vi "process vision.vi"(8 "?":errorcluster, 11 "Processed Image":T1(plugin-control)) -> (2 "Annotated Image Out":T1(plugin-control), 3 "Processed Image Out":T1(plugin-control))   [LabVIEW 2015]
uses:
  <vilib>/vision/NI_Vision_Development_Module.lvlib
panel:
  out "output cluster":cluster{dbl[], dbl[], dbl[]}
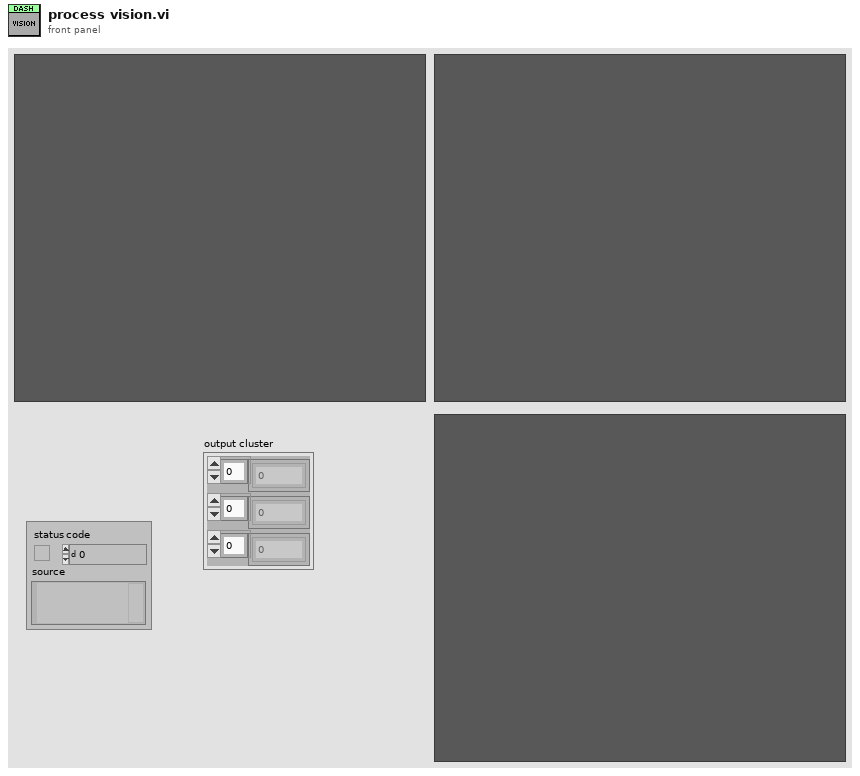
[diagram p1: front panel]
types:
  T1 = typedef "IMAQ Image.ctl" = refnum<image>
  T2 = typedef "Image Type" = u32
  T3 = cluster{"Desired Font (Application)":enum16{"User-specified Font", "Application Font", "System Font", "Dialog Font"}, "[User-specified Font]":cluster{"Font Name":string, "Size":i16, "Strikeout?":bool, "Italic?":bool, "Underline?":bool, "Outline?":bool, "Shadow?":bool, "Bold?":bool, "Rotation Angle":dbl}, "Horizontal Alignment":i16, "Vertical Alignment":i16}
  T4 = cluster{"Left":i32, "Top":i32, "Right":i32, "Bottom":i32}
  T5 = cluster{"Area":dbl, "Number of Holes":dbl, "Bounding Rect":cluster{"Left":dbl, "Top":dbl, "Right":dbl, "Bottom":dbl}, "Center of Mass":cluster{"X":dbl, "Y":dbl}, "Orientation":dbl, "Dimensions":cluster{"Width":dbl, "Height":dbl}}[]
  T6 = cluster{"Left":dbl, "Top":dbl, "Right":dbl, "Bottom":dbl}
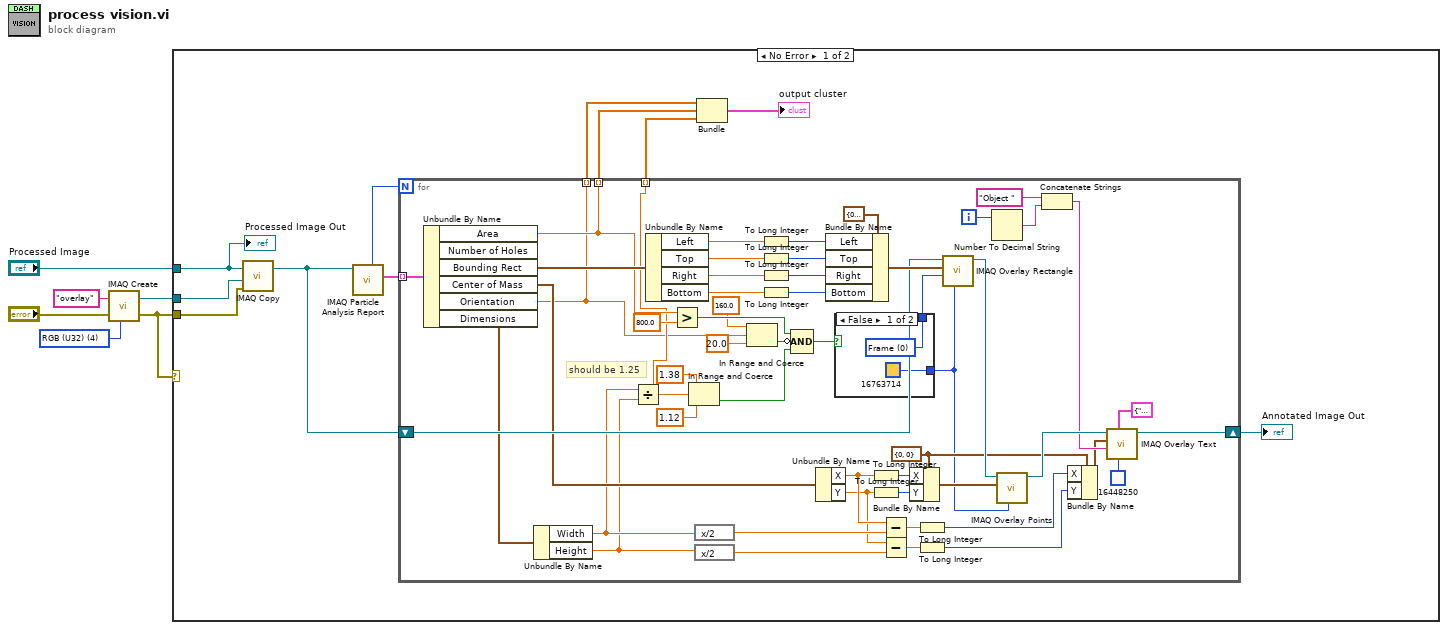
[diagram p0: block diagram]
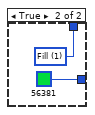
[diagram p2: hidden frame]
diagram:
  w2 = T2 4 items=["Grayscale (U8)", "Grayscale (I16)", "Grayscale (SGL)", "Complex (CSG)", "RGB (U32)", "HSL (U32)", "RGB (U64)", "Grayscale (U16)"] ("Image Type")
  n1 = call "IMAQ Create"("Image Name"="overlay", "Image Type"=w2, "error in (no error)"="?") -> ("New Image"=w5:T1, "error out"=w1:errorcluster)  [unwired: 2 in]
  n2 = case shown="No Error" w1 {
    tunnel: w5 -> [w14 _]
    tunnel: "Processed Image" -> [w12 _]
    tunnel: w1 -> [w11 _]
    frame No Error {
      n3 = call "IMAQ Copy"("error in (no error)"=w11, "Image Dst"=w14, "Image Src"=w12) -> ("Image Dst Out"=w13:T1)  [unwired: 3 in, 1 out]
      n4 = call "IMAQ Particle Analysis Report"("Image"=w13) -> ("Particle Reports (Pixels)"=w16:T5, "Number of Particles"=w17:i32)  [unwired: 5 in, 4 out]
      n5 = for {
        N: w17 -> [_]
        tunnel: w16 -> [w70] mode=indexing
        shift-right: [w52] -> w15
        shift-left: w13 -> [w59]
        tunnel: [w20] -> w10 mode=indexing
        tunnel: [w23] -> w9 mode=indexing
        tunnel: [w22] -> w8 mode=indexing
        i -> [w48]
        w45 = cluster{"X":i32, "Y":i32} {"X"=0, "Y"=0} ("Point")
        # "should be 1.25"
        n6 = Unbundle By Name(w70) -> ("Area"=w23:dbl, "Bounding Rect"=w69:T6, "Center of Mass"=w58:cluster{"X":dbl, "Y":dbl}, "Orientation"=w20:dbl, "Dimensions"=w44:cluster{"Width":dbl, "Height":dbl})  [unwired: 1 out]
        n7 = Unbundle By Name(w44) -> ("Width"=w36:dbl, "Height"=w35:dbl)
        n8 = Divide(x=w36, y=w35) -> (x/y=w22:dbl)
        n9 = Unbundle By Name(w69) -> ("Left"=w67:dbl, "Top"=w65:dbl, "Right"=w61:dbl, "Bottom"=w28:dbl)
        n10 = Greater?(x=w23, y=800.0) -> (0:w26:bool)
        n11 = In Range and Coerce(upper limit=1.38, x=w22, lower limit=1.12 ("upper limit")) -> (In Range?=w32:bool)  [unwired: 1 out]
        n12 = expression code="x/2"(w36) -> (w43:dbl)
        n13 = expression code="x/2"(w35) -> (w39:dbl)
        n14 = In Range and Coerce(upper limit=160.0, x=w20, lower limit=20.0 ("y")) -> (In Range?=w21:bool)  [unwired: 1 out]
        n15 = To Long Integer(number=w67) -> (32bit integer=w66:i32)
        n16 = To Long Integer(number=w65) -> (32bit integer=w64:i32)
        n17 = To Long Integer(number=w61) -> (32bit integer=w63:i32)
        n18 = To Long Integer(number=w28) -> (32bit integer=w62:i32)
        n19 = Compound Arithmetic op=AND(w26, invert w21, w32) -> (w30:bool)
        n20 = Unbundle By Name(w58) -> ("X"=w25:dbl, "Y"=w24:dbl)
        n21 = Bundle By Name(cluster=T4 {"Left"=0, "Top"=0, "Right"=0, "Bottom"=0} ("Rectangle"), "Left"=w66, "Top"=w64, "Right"=w63, "Bottom"=w62) -> (w60:T4)
        n22 = case shown="False" w30 {
          tunnel: [u32 16763714 ("Color") u32 56381 ("Color")] -> w31
          tunnel: [w71 w73] -> w29
          frame False {
            w71 = u32 0 items=["Frame", "Fill", "Highlight"] ("Drawing Mode (Frame)")
          }
          frame True {
            w73 = u32 1 items=["Frame", "Fill", "Highlight"] ("Drawing Mode (Frame)")
          }
        }
        n23 = To Long Integer(number=w25) -> (32bit integer=w56:i32)
        n24 = To Long Integer(number=w24) -> (32bit integer=w57:i32)
        n25 = Subtract(x=w25, y=w43) -> (x-y=w42:dbl)
        n26 = Subtract(x=w24, y=w39) -> (x-y=w40:dbl)
        n27 = Bundle By Name(cluster=w45, "X"=w56, "Y"=w57) -> (w55:cluster{"X":i32, "Y":i32})
        n28 = To Long Integer(number=w42) -> (32bit integer=w41:i32)
        n29 = To Long Integer(number=w40) -> (32bit integer=w38:i32)
        n30 = call "IMAQ Overlay Rectangle"("Color"=w31, "Drawing Mode (Frame)"=w29, "Rectangle"=w60, "Image"=w59) -> ("Image Out"=w54:T1)  [unwired: 6 in, 1 out]
        n31 = Number To Decimal String(number=w48) -> (decimal integer string=w49:string)  [unwired: 1 in]
        n32 = call "IMAQ Overlay Points"("Color"=w31, "Point"=w55, "Image"=w54) -> ("Image Out"=w53:T1)  [unwired: 7 in, 1 out]
        n33 = Concatenate Strings("Object " ("String"), w49) -> (w47:string)
        n34 = Bundle By Name(cluster=w45, "X"=w41, "Y"=w38) -> (w46:cluster{"X":i32, "Y":i32})
        n35 = call "IMAQ Overlay Text"("Text Color (black)"=u32 16448250 ("Color"), "Font, Size & Style"=T3 {"Desired Font (Application)"=enum."User-specified Font", "[User-specified Font]"={"Font Name"="Roboto Light", "Size"=12, "Strikeout?"=FALSE, "Italic?"=FALSE, "Underline?"=FALSE, "Outline?"=FALSE, "Shadow?"=FALSE, "Bold?"=FALSE, "Rotation Angle"=0.0}, "Horizontal Alignment"=0, "Vertical Alignment"=0}, "String"=w47, "Origin"=w46, "Image"=w53) -> ("Image Out"=w52:T1)  [unwired: 5 in, 1 out]
      }
      "Annotated Image Out" <- w15
      n36 = Bundle(w10, w9, w8) -> (→"output cluster":cluster{dbl[], dbl[], dbl[]})  [unwired: 1 in]
      "Processed Image Out" <- w12
    }
    frame Error {
    }
  }
